vi "Set Spool.vi"(7 "framebuffersize":i32, 9 "path":string, 10 "method":i32, 11 "active":i32) -> (1 "path out":string, 3 "function return":u32)   [LabVIEW 2018, in "AndorSDK.lvlib"]
doc: "EXPNETTYPE unsigned int WINAPI SetSpool(int active, int method, char * path, int framebuffersize);"
uses:
  AndorSDK.lvlib
  ATMCD32D.dll
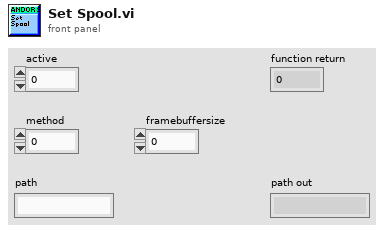
[diagram p1: front panel]
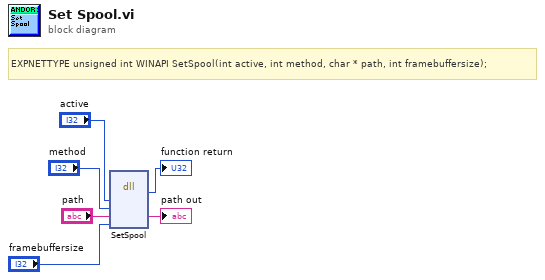
[diagram p0: block diagram]
diagram:
  # "EXPNETTYPE unsigned int WINAPI SetSpool(int active, int method, char * path, int framebuffersize);"
  n1 = dll-call lib="PTH2babs E\nPersönliches02 - Arbeit03-HiwijobsLabviewCodelibANDOR\tAndor SDK\nATMCD32D.*" fn="SetSpool"("active"="active", "method"="method", "path"="path", "framebuffersize"="framebuffersize") -> (→"function return":u32, "path"=→"path out":string)  [unwired: 6 in, 2 out]
